vi "FS Operation.vi"   [LabVIEW 2019]
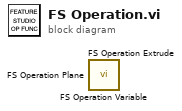
[diagram p0: block diagram]
diagram:
  n1 = call <userlib>:"FS Operation Variable.vi"() -> ()  [unwired: 11 in, 1 out]
  n2 = call <userlib>:"FS Operation Extrude.vi"() -> ()  [unwired: 11 in, 1 out]
  n3 = call <userlib>:"FS Operation Plane.vi"() -> ()  [unwired: 11 in, 1 out]
